vi "Read Wait(ms).vi"(8 "error in (no error)":errorcluster, 11 "Protocol Interface in":refnum<class "Protocol Interface.lvclass">) -> (0 "error out":errorcluster, 2 "Wait(ms)":dbl, 3 "Protocol Interface out":refnum<class "Protocol Interface.lvclass">)   [LabVIEW 2018, in "Protocol Interface.lvlib" / "Protocol Interface.lvclass"]
uses:
  Protocol Interface.lvclass
  Protocol Interface.lvclass/Protocol Interface.ctl
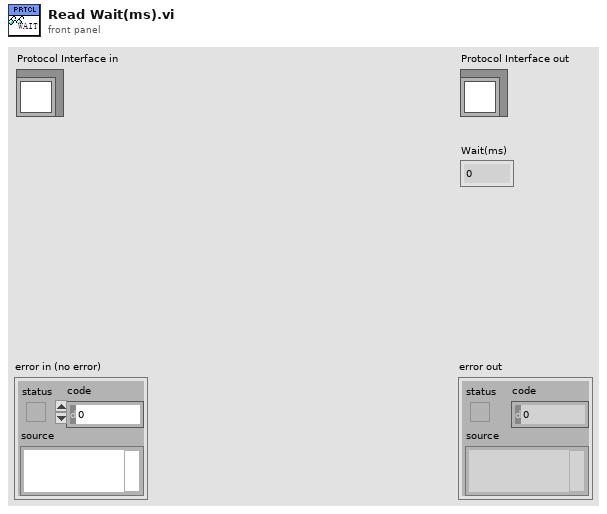
[diagram p1: front panel]
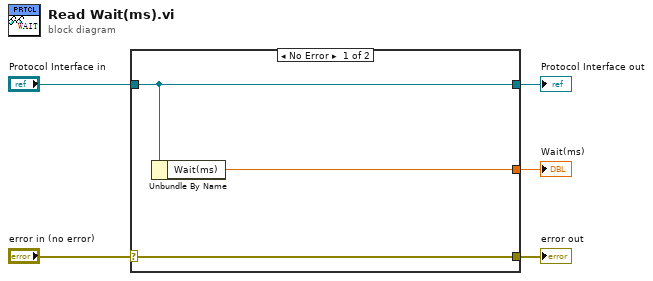
[diagram p0: block diagram]
diagram:
  n1 = case shown="No Error" "error in (no error)" {
    selector: "error in (no error)" -> [w8 w9]
    tunnel: [w8 w9] -> w4
    tunnel: [w7 w10] -> w2
    tunnel: "Protocol Interface in" -> [w7 w10]
    tunnel: [w6 _] -> w1
    frame No Error {
      n2 = Unbundle By Name(w7) -> ("Wait(ms)"=w6:dbl)
    }
    frame Error {
    }
  }
  "error out" <- w4
  "Protocol Interface out" <- w2
  "Wait(ms)" <- w1
